vi "AOA estimation using MIMO prototyping system channel state information.vi"() -> ()   [LabVIEW 2015]
uses:
  <vilib>/Native 3D Graph/xcontrol/3DPC_SurfacePlot.xctl
  <vilib>/Analysis/1siggen.llb/Ramp Pattern by Samples.vi
  <vilib>/Utility/file.llb/Read Delimited Spreadsheet (DBL).vi
  <vilib>/Analysis/1siggen.llb/Ramp Pattern by Delta.vi
  <vilib>/Analysis/NI_AALBase.lvlib
panel:
  out "Elevation angle":dbl format="%#_g (deg)"
  out "Azimuth":dbl format="%#_g (deg)"
  out "Element RP":refnum<class "Base Datatype.lvclass">[](xcontrol)
  out "Array RP":refnum<class "Base Datatype.lvclass">[](xcontrol)
  in  "VERT 2450 Pattern":dbl[][](array[numeric])=array361x361[130321 elements]
  out "YZ X=0":cluster{dbl[], dbl[]}(graph)
  out "XZ Y=0":cluster{dbl[], dbl[]}(graph)
  out "XY Z=0":cluster{dbl[], dbl[]}(graph)
  in  "stop":bool
  out "Overall RP":refnum<class "Base Datatype.lvclass">[](xcontrol)
  in  "Dy":dbl=0.045 format="%#_g (m)"
  out "Phase y":dbl[](array[numeric]) format="%#_g  (rad)"
  out "Amplitude Y":dbl[](array[numeric])=[1.0, 1.0, 1.0, 1.0, 1.0, 1.0, 1.0, 1.0, 1.0, 1.0, 1.0, 1.0, 1.0, 1.0, 1.0, 1.0] format="%#_g (V)"
  in  "Wavelength":dbl=0.136 format="%#_g (m)"
  in  "Dx":dbl=0.05 format="%#_g (m)"
  out "Phase X":dbl[](array[numeric]) format="%#_g (rad)"
  out "Amplitude X":dbl[](array[numeric])=[1.0, 1.0, 1.0, 1.0, 1.0, 1.0, 1.0, 1.0, 1.0, 1.0, 1.0, 1.0, 1.0, 1.0, 1.0, 1.0] format="%#_6g (V)"
  # "MS signal AOA estimation results"
  # "Anntenna arrangement"
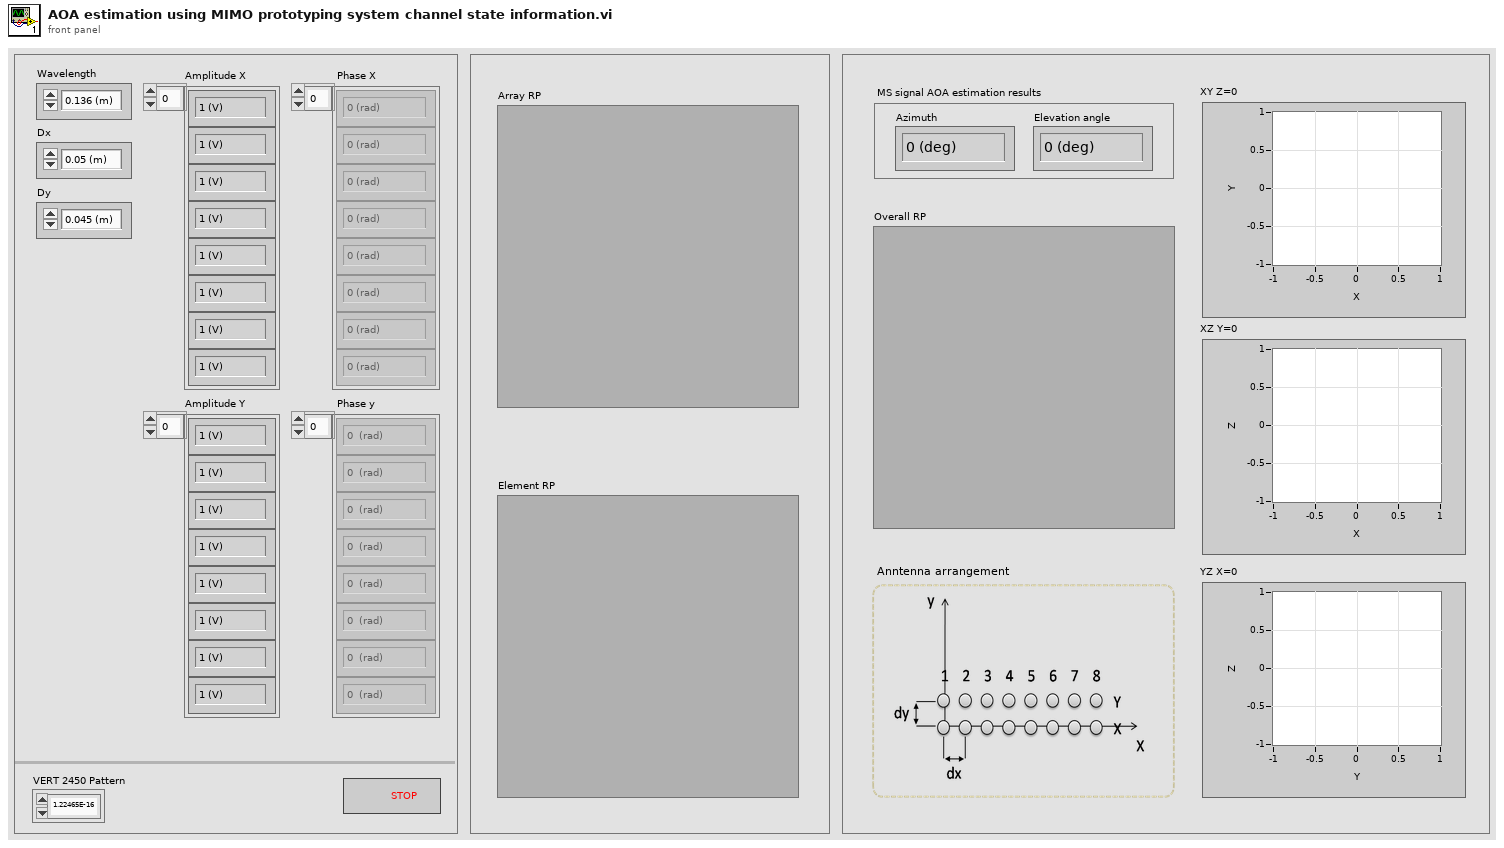
[diagram p1: front panel]
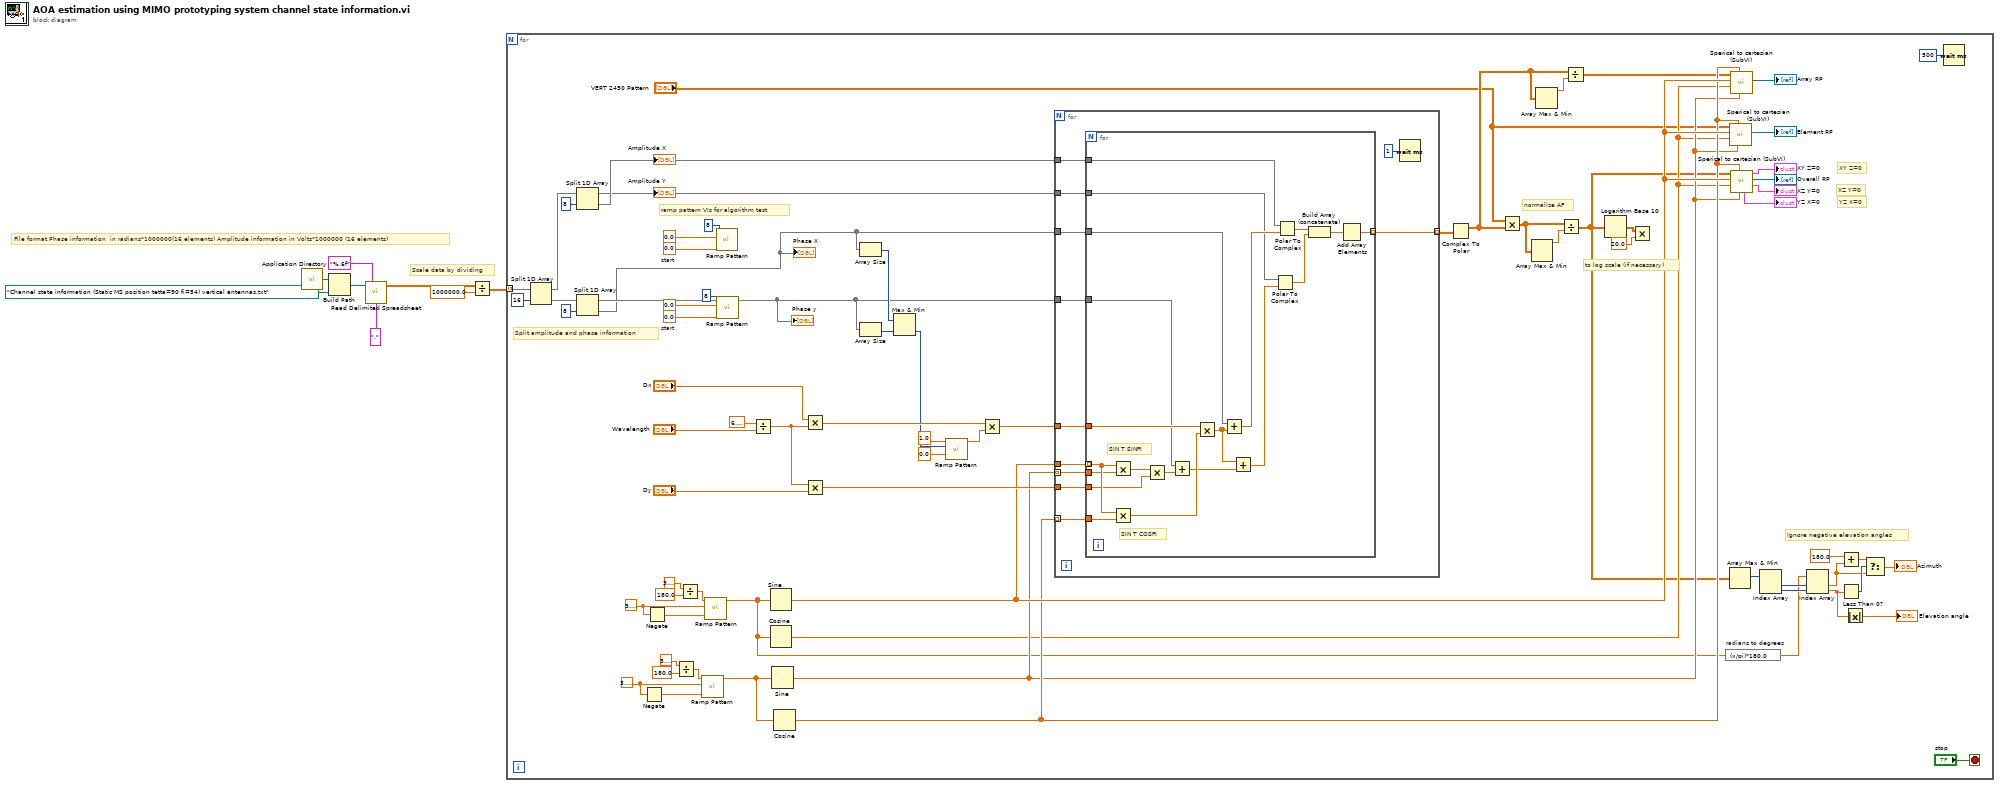
[diagram p0: block diagram]
diagram:
  # "File format Phase information  in radians*1000000(16 elements) Amplitude information in Volts*1000000 (16 elements)"
  # "Scale data by dividing"
  n1 = call <vilib>:"Application Directory.vi"() -> ("Application Directory"=w2:path)
  n2 = Build Path(base path=w2, name or relative path=path "Channel state information (Static MS position tetta=90 fi=54) vertical antennas.txt" ("file path (dialog if empty)")) -> (appended path=w3:path)
  n3 = call-poly <vilib>:"Read Delimited Spreadsheet.vi"("file path (dialog if empty)"=w3, "format (%.3f)"="%.6f", "delimiter (\\t)"="," ("delimiter (\\t)")) -> ("all rows"=w5:dbl[][])  [unwired: 7 in, 5 out]
  n4 = Divide(x=w5, y=1000000.0) -> (x/y=w6:dbl[][])
  n5 = for {
    tunnel: w6 -> [w33] mode=indexing
    stop <- "stop" stop-if-true
    w58 = 3.141592653589793
    w66 = 0.0  # start
    w72 = 0.0  # start
    w57 = 3.141592653589793
    # "Ignore negative elevation angles"
    # "normalize AF"
    # "to log scale (if necessary)"
    # "ramp pattern VIs for algorithm test"
    # "Split amplitude and phase information"
    # "YZ X=0"
    # "XZ Y=0"
    # "XY Z=0"
    n6 = Split 1D Array(array=w33, index=16) -> (first subarray=w30:dbl[], second subarray=w28:dbl[])
    n7 = Split 1D Array(array=w30, index=8) -> (first subarray=w25:dbl[], second subarray=w26:dbl[])
    "Amplitude X" <- w26
    "Amplitude Y" <- w25
    n8 = Split 1D Array(array=w28, index=8) -> (first subarray=w24:dbl[], second subarray=w23:dbl[])
    "Phase X" <- w23
    "Phase y" <- w24
    n9 = Negate(x=w58) -> (-x=w59:dbl)
    n10 = Negate(x=w57) -> (-x=w60:dbl)
    n11 = Divide(x=3.141592653589793, y=180.0) -> (x/y=w64:dbl)
    n12 = Divide(x=3.141592653589793, y=180.0) -> (x/y=w75:dbl)
    n13 = call-poly <vilib>:"Ramp Pattern.vi"("start"=w59, "end"=w58, "delta"=w64) -> ("Ramp Pattern"=w19:dbl[])  [unwired: 6 in, 2 out]
    n14 = call-poly <vilib>:"Ramp Pattern.vi"("start"=w60, "end"=w57, "delta"=w75) -> ("Ramp Pattern"=w17:dbl[])  [unwired: 6 in, 2 out]
    n15 = call-poly <vilib>:"Ramp Pattern.vi"("start"=w72, "end"=0.0 ("PhaseX"), "samples"=8) -> ()  [unwired: 7 in, 2 out]
    n16 = call-poly <vilib>:"Ramp Pattern.vi"("start"=w66, "end"=0.0 ("PhaseY"), "samples"=8) -> ()  [unwired: 7 in, 2 out]
    n17 = Divide(x=6.283185307179586, y="Wavelength") -> (x/y=w69:dbl)
    n18 = Sine(x=w17) -> (sin(x)=w45:dbl[])
    n19 = Cosine(x=w17) -> (cos(x)=w38:dbl[])
    n20 = Sine(x=w19) -> (sin(x)=w39:dbl[])
    n21 = Cosine(x=w19) -> (cos(x)=w44:dbl[])
    n22 = Multiply(x="Dx", y=w69) -> (x*y=w78:dbl)
    n23 = Multiply(x=w69, y="Dy") -> (x*y=w61:dbl)
    n24 = Array Size(array=w23) -> (size(s)=w48:i32)
    n25 = Array Size(array=w24) -> (size(s)=w49:i32)
    n26 = Max & Min(x=w48, y=w49) -> (min(x,y)=w47:i32)  [unwired: 1 out]
    n27 = call-poly <vilib>:"Ramp Pattern.vi"("start"=0.0, "end"=w47, "delta"=1.0 ("start")) -> ("Ramp Pattern"=w79:dbl[])  [unwired: 6 in, 2 out]
    n28 = Multiply(x=w78, y=w79) -> (x*y=w74:dbl[])
    n29 = for {
      tunnel: w45 -> [w94]
      tunnel: w74 -> [w93]
      tunnel: w26 -> [w92]
      tunnel: w23 -> [w91]
      tunnel: [w85] -> w53 mode=indexing
      tunnel: w24 -> [w90]
      tunnel: w39 -> [w88] mode=indexing
      tunnel: w44 -> [w89] mode=indexing
      tunnel: w61 -> [w87]
      tunnel: w25 -> [w86]
      n30 = for {
        tunnel: w94 -> [w110] mode=indexing
        tunnel: w93 -> [w113]
        tunnel: w92 -> [w114]
        tunnel: w91 -> [w105]
        tunnel: [w112] -> w85 mode=indexing
        tunnel: w90 -> [w101]
        tunnel: w89 -> [w111]
        tunnel: w88 -> [w109]
        tunnel: w87 -> [w102]
        tunnel: w86 -> [w99]
        # "SIN T COSFI"
        # "SIN T SINFI"
        n31 = Multiply(x=w110, y=w109) -> (x*y=w108:dbl)
        n32 = Multiply(x=w110, y=w111) -> (x*y=w107:dbl)
        n33 = Multiply(x=w108, y=w102) -> (x*y=w106:dbl)
        n34 = Add(x=w101, y=w106) -> (x+y=w104:dbl[])
        n35 = Multiply(x=w113, y=w107) -> (x*y=w100:dbl[])
        n36 = Add(x=w105, y=w100) -> (x+y=w103:dbl[])
        n37 = Add(x=w100, y=w104) -> (x+y=w98:dbl[])
        n38 = Polar To Complex(1:w98, 2:w99) -> (0:w97:cdb[])
        n39 = Polar To Complex(1:w103, 2:w114) -> (0:w96:cdb[])
        n40 = Build Array (concatenate)(w96, w97) -> (w95:cdb[])
        n41 = Add Array Elements(numeric array=w95) -> (sum=w112:cdb)
      }
      n42 = Wait (ms)(milliseconds to wait=u32 1) -> ()  [unwired: 1 out]
    }
    n43 = Complex To Polar(r * e^(i*theta)=w53) -> (r=w36:dbl[][])  [unwired: 1 out]
    n44 = Multiply(x="VERT 2450 Pattern", y=w36) -> (x*y=w51:dbl[][])
    n45 = Array Max & Min(array=w51) -> (max value=w56:dbl)  [unwired: 3 out]
    n46 = Array Max & Min(array=w36) -> (max value=w37:dbl)  [unwired: 3 out]
    n47 = Divide(x=w51, y=w56) -> (x/y=w22:dbl[][])
    n48 = Divide(x=w36, y=w37) -> (x/y=w35:dbl[][])
    n49 = Logarithm Base 10(1:w22) -> (0:w55:dbl[][])
    n50 = Multiply(x=w55, y=20.0) -> ()  [unwired: 1 out]
    n51 = expression code="(x/pi)*180.0" "radians to degrees"(w17) -> (w16:dbl[])
    n52 = Array Max & Min(array=w22) -> (max index (indices)=w21:i32[])  [unwired: 3 out]
    n53 = call "Sperical to cartesian (SubVI).vi"("SinFI"=w39, "Cos FI"=w44, "Cos Tetta"=w38, "SinTetta"=w45, "Data"="VERT 2450 Pattern") -> ("plots out"=→"Element RP":refnum<class "Base Datatype.lvclass">[])  [unwired: 3 in, 3 out]
    n54 = call "Sperical to cartesian (SubVI).vi"("SinFI"=w39, "Cos FI"=w44, "Cos Tetta"=w38, "SinTetta"=w45, "Data"=w35) -> ("plots out"=→"Array RP":refnum<class "Base Datatype.lvclass">[])  [unwired: 3 in, 3 out]
    n55 = call "Sperical to cartesian (SubVI).vi"("SinFI"=w39, "Cos FI"=w44, "Cos Tetta"=w38, "SinTetta"=w45, "Data"=w22) -> ("XZ"=→"XZ Y=0":cluster{dbl[], dbl[]}, "plots out"=→"Overall RP":refnum<class "Base Datatype.lvclass">[], "XY3"=→"XY Z=0":cluster{dbl[], dbl[]}, "YZ"=→"YZ X=0":cluster{dbl[], dbl[]})  [unwired: 3 in]
    n56 = Index Array(array=w21) -> (element #1=w20:i32, element #2=w18:i32)  [unwired: 2 in]
    n57 = Index Array(array=w16, index #1=w20, index #2=w18) -> (element #1=w10:dbl, element #2=w13:dbl)
    n58 = Add(x=180.0, y=w10) -> (x+y=w11:dbl)
    n59 = Less Than 0?(x=w13) -> (x < 0?=w12:bool)
    n60 = Absolute Value(x=w13) -> (abs(x)=→"Elevation angle":dbl)
    n61 = Select(t=w11, s=w12, f=w10) -> (s? t:f=→"Azimuth":dbl)
    n62 = Wait (ms)(milliseconds to wait=u32 500) -> ()  [unwired: 1 out]
  }
